vi "Traffic light.vi"() -> ()   [LabVIEW 2018]
panel:
  out "Boolean 3":bool
  out "Boolean 2":bool
  out "Boolean":bool
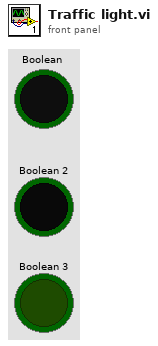
[diagram p1: front panel]
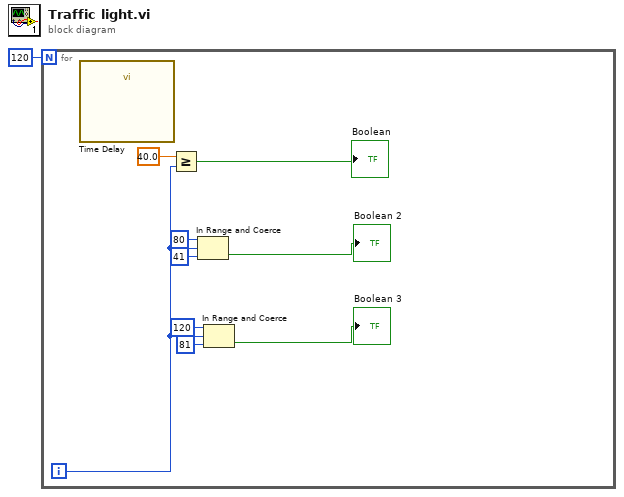
[diagram p0: block diagram]
diagram:
  n1 = for {
    N: 120 -> [_]
    i -> [w5]
    n2 = call "Time Delay"() -> ()  [unwired: 11 in, 1 out]
    n3 = Greater Or Equal?(x=40.0, y=w5) -> (x >= y?=→"Boolean":bool)
    n4 = In Range and Coerce(upper limit=80, x=w5, lower limit=41) -> (In Range?=→"Boolean 2":bool)  [unwired: 1 out]
    n5 = In Range and Coerce(upper limit=120, x=w5, lower limit=81) -> (In Range?=→"Boolean 3":bool)  [unwired: 1 out]
  }
